vi "KProp-Table to Arg List.vi"(0 "Rows":T1[](array[typedef]), 7 "type":string) -> (8 "Args":string[](array[string]))   [LabVIEW 2020, in "KPropertyTable.xctl"]
uses:
  KPropertyTable.xctl
  RowData.ctl
  DataType.ctl
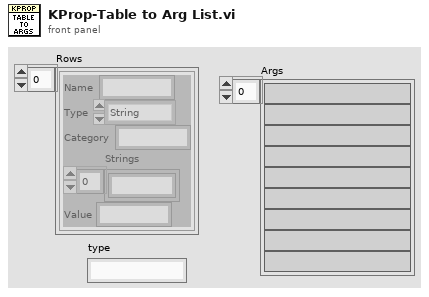
[diagram p1: front panel]
types:
  T1 = typedef "KPropertyTable.xctl/RowData.ctl" = cluster{"Name":string, "Type":T2, "Category":string, "Strings":string[], "Value":string}
  T2 = typedef "KPropertyTable.xctl/DataType.ctl" = enum16{"String", "Enum", "Int", "Double", "Boolean", "Ring", "Formula"}
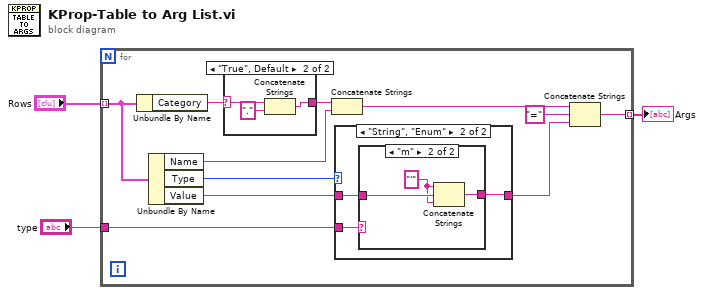
[diagram p0: block diagram]
diagram:
  n1 = for {
    tunnel: "Rows" -> [w14] mode=indexing
    tunnel: [w6] -> w2 mode=indexing
    tunnel: "type" -> [w4]
    n2 = Unbundle By Name(w14) -> ("Category"=w13:string)
    n3 = Unbundle By Name(w14) -> ("Name"=w11:string, "Type"=w10:T2, "Value"=w9:string)
    n4 = case shown="\"True\", Default" w13 {
      selector: w13 -> [w15 w18]
      tunnel: [w15 w17] -> w12
      frame "" {
      }
      frame "True", Default {
        n5 = Concatenate Strings(w18, "." ("string")) -> (w17:string)
      }
    }
    n6 = Concatenate Strings(w12, w11) -> (w8:string)
    n7 = case shown="\"String\", \"Enum\"" w10 {
      tunnel: w9 -> [w19 w21]
      tunnel: [w19 w20] -> w5
      tunnel: w4 -> [_ w22]
      frame "Int", Default {
      }
      frame "String", "Enum" {
        n8 = case shown="\"m\"" w22 {
          tunnel: w21 -> [w23 w26]
          tunnel: [w23 w24] -> w20
          frame "False", Default {
          }
          frame "m" {
            w25 = "'"
            n9 = Concatenate Strings(w25, w26, w25) -> (w24:string)
          }
        }
      }
    }
    n10 = Concatenate Strings(w8, "=" ("string"), w5) -> (w6:string)
  }
  "Args" <- w2
